vi "MultiTool-Track-Generate-ndipolarisFileOutput-Q-vectors-Accepts Joystick Command with Time Display-Testing time diff with tick-26Apr2017.vi"() -> ()   [LabVIEW 2013]
panel:
  out "TIME":string
  out "bytes written":i32
  out "Return time string":string
  out "Length":u8
  out "Command":u8
  out "Tool 2":T1={"Port Handle"="", "Frame Number"=0, "Tx"=0.0, "Ty"=0.0, "Tz"=0.0, "Q0"=0.0, "Qx"=0.0, "Qy"=0.0, "Qz"=0.0, "Deviation"=0.0, " Markers Missing"=TRUE, "Out of Volume"=TRUE} {"Deviation" format="%#.4f"; "Qz" format="%#.4f"; "Qy" format="%#.4f"; "Qx" format="%#.4f"; "Q0" format="%#.4f"; "Tz" format="%#.2f"; "Ty" format="%#.2f"; "Tx" format="%#.2f"}
  in  "Location of ROM File for Tool 2":path=path "C:/Program Files (x86)/Northern Digital Inc/8700339.rom"
  in  "NDI  Running":bool=TRUE
  out "Stop Reading":bool=TRUE
  out "Start Reading":bool
  out "Object Identifier":string="0"
  in  "Track Outside Measurement Volume? (F:No)":bool
  in  "Track Stray Markers? (F:No)":bool
  out "Tool 1":T1={"Port Handle"="", "Frame Number"=0, "Tx"=0.0, "Ty"=0.0, "Tz"=0.0, "Q0"=0.0, "Qx"=0.0, "Qy"=0.0, "Qz"=0.0, "Deviation"=0.0, " Markers Missing"=TRUE, "Out of Volume"=TRUE} {"Deviation" format="%#.4f"; "Qz" format="%#.4f"; "Qy" format="%#.4f"; "Qx" format="%#.4f"; "Q0" format="%#.4f"; "Tz" format="%#.2f"; "Ty" format="%#.2f"; "Tx" format="%#.2f"}
  out "TCP loop":i32
  in  "TCP Server Running":bool=TRUE
  in  "Output Directory":path=path "C:/Users/Diogo/Desktop/NDI-Labview Gripper"
  out "NDI Loop":i32
  in  "VISA resource name":refnum<visa-resource-name>="COM8"
  in  "Reset? (T:Yes)":bool=TRUE
  in  "Location of ROM File for Tool 1":path=path "C:/Program Files (x86)/Northern Digital Inc/8700449.rom"
  in  "Serial Configuration":T2={"Baud Rate (9600)"=9600, "Flow Control (0:None)"=0, "Parity"=0, "Data Bits"=8, "Stop Bits"=10} {"Stop Bits" items=["1.0"=10, "2.0"=20]; "Parity" items=["None", "Odd", "Even"]; "Flow Control (0:None)" items=["None", "XON/XOFF"]; "Baud Rate (9600)" items=["9600"=9600, "14.4k"=14400, "19.2k"=19200, "38.4k"=38400, "57.6k "=57600, "115.2k"=115200]}
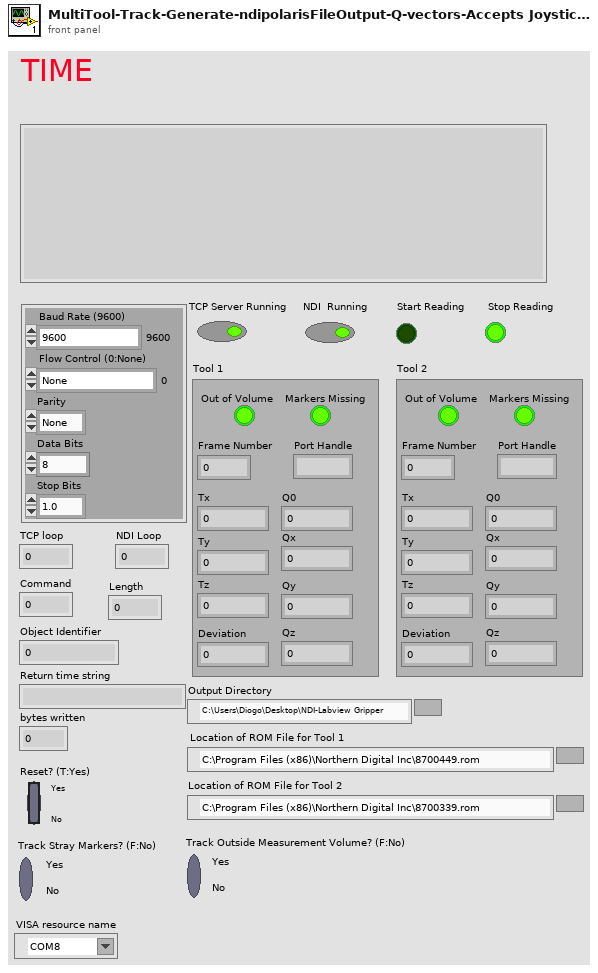
[diagram p1: front panel]
types:
  T1 = cluster{"Port Handle":string, "Frame Number":i32, "Tx":dbl, "Ty":dbl, "Tz":dbl, "Q0":dbl, "Qx":dbl, "Qy":dbl, "Qz":dbl, "Deviation":dbl, " Markers Missing":bool, "Out of Volume":bool}
  T2 = cluster{"Baud Rate (9600)":u32, "Flow Control (0:None)":u16, "Parity":u16, "Data Bits":u16, "Stop Bits":u16}
  T3 = cluster{"Port Handle":string, "Frame Number":u32, "Tx":dbl, "Ty":dbl, "Tz":dbl, "Q0":dbl, "Qx":dbl, "Qy":dbl, "Qz":dbl, "Deviation":dbl, "Missing?":bool, "Out of Volume?":bool}[]
  T4 = cluster{"Transformations[0]":cluster{"Port Handle":string, "Frame Number":u32, "Tx":dbl, "Ty":dbl, "Tz":dbl, "Q0":dbl, "Qx":dbl, "Qy":dbl, "Qz":dbl, "Deviation":dbl, "Missing?":bool, "Out of Volume?":bool}, "Transformations[1]":cluster{"Port Handle":string, "Frame Number":u32, "Tx":dbl, "Ty":dbl, "Tz":dbl, "Q0":dbl, "Qx":dbl, "Qy":dbl, "Qz":dbl, "Deviation":dbl, "Missing?":bool, "Out of Volume?":bool}, "Transformations[2]":cluster{"Port Handle":string, "Frame Number":u32, "Tx":dbl, "Ty":dbl, "Tz":dbl, "Q0":dbl, "Qx":dbl, "Qy":dbl, "Qz":dbl, "Deviation":dbl, "Missing?":bool, "Out of Volume?":bool}, "Transformations[3]":cluster{"Port Handle":string, "Frame Number":u32, "Tx":dbl, "Ty":dbl, "Tz":dbl, "Q0":dbl, "Qx":dbl, "Qy":dbl, "Qz":dbl, "Deviation":dbl, "Missing?":bool, "Out of Volume?":bool}, "Transformations[4]":cluster{"Port Handle":string, "Frame Number":u32, "Tx":dbl, "Ty":dbl, "Tz":dbl, "Q0":dbl, "Qx":dbl, "Qy":dbl, "Qz":dbl, "Deviation":dbl, "Missing?":bool, "Out of Volume?":bool}, "Transformations[5]":cluster{"Port Handle":string, "Frame Number":u32, "Tx":dbl, "Ty":dbl, "Tz":dbl, "Q0":dbl, "Qx":dbl, "Qy":dbl, "Qz":dbl, "Deviation":dbl, "Missing?":bool, "Out of Volume?":bool}, "Transformations[6]":cluster{"Port Handle":string, "Frame Number":u32, "Tx":dbl, "Ty":dbl, "Tz":dbl, "Q0":dbl, "Qx":dbl, "Qy":dbl, "Qz":dbl, "Deviation":dbl, "Missing?":bool, "Out of Volume?":bool}, "Transformations[7]":cluster{"Port Handle":string, "Frame Number":u32, "Tx":dbl, "Ty":dbl, "Tz":dbl, "Q0":dbl, "Qx":dbl, "Qy":dbl, "Qz":dbl, "Deviation":dbl, "Missing?":bool, "Out of Volume?":bool}, "Transformations[8]":cluster{"Port Handle":string, "Frame Number":u32, "Tx":dbl, "Ty":dbl, "Tz":dbl, "Q0":dbl, "Qx":dbl, "Qy":dbl, "Qz":dbl, "Deviation":dbl, "Missing?":bool, "Out of Volume?":bool}}
  T5 = cluster{"Port Handle":string, "Frame Number":u32, "Tx":dbl, "Ty":dbl, "Tz":dbl, "Q0":dbl, "Qx":dbl, "Qy":dbl, "Qz":dbl, "Deviation":dbl, "Missing?":bool, "Out of Volume?":bool}
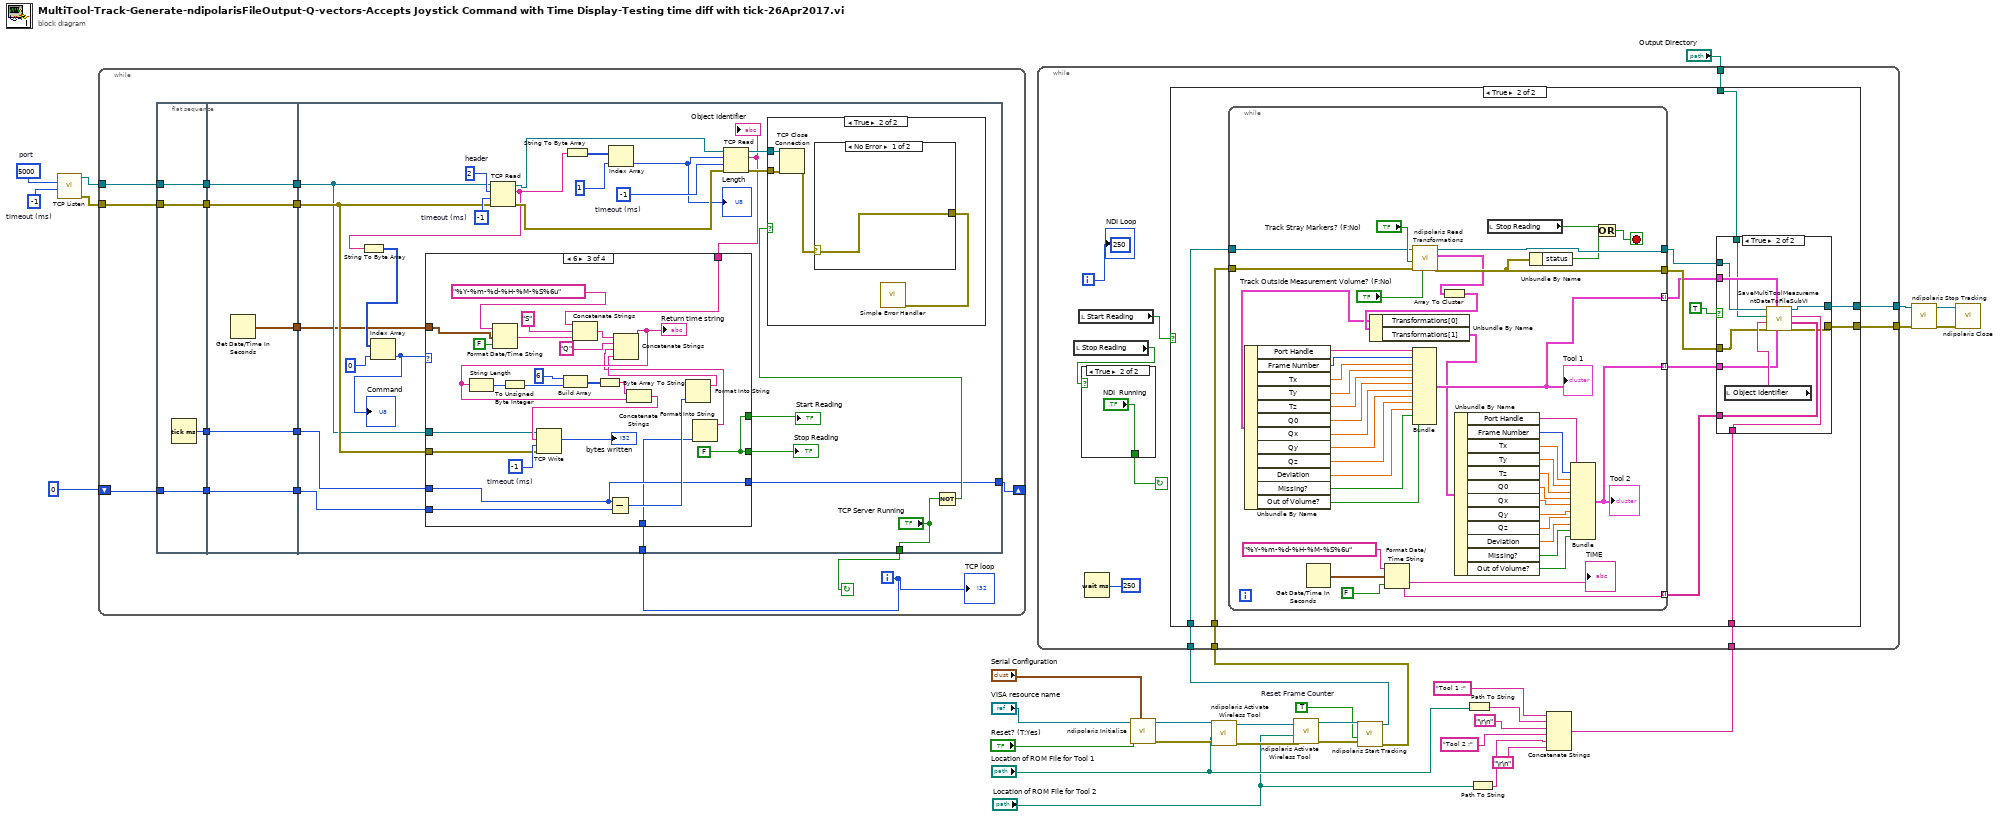
[diagram p0: block diagram]
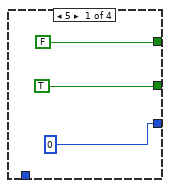
[diagram p2: hidden frame]
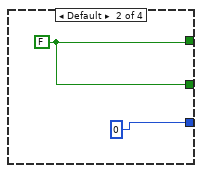
[diagram p3: hidden frame]
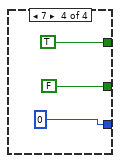
[diagram p4: hidden frame]
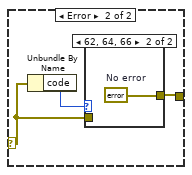
[diagram p6: hidden frame]
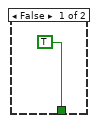
[diagram p8: hidden frame]
diagram:
  w22 = TRUE  # Reset Frame Counter
  w31 = u16 5000  # port
  w30 = i8 -1  # timeout (ms)
  n1 = call <vilib>:"TCP Listen.vi"("timeout ms (wait forever: -1)"=w30, "port"=w31) -> ("error out"=w25:errorcluster, "connection ID"=w26:refnum<k5>)  [unwired: 5 in, 3 out]
  n2 = while {
    tunnel: w26 -> [w44]
    tunnel: w25 -> [w45]
    shift-right: [w38] -> _
    shift-left: u32 0 -> [w40]
    i -> [w32]
    stop <- w46 continue-if-true
    n3 = flat-sequence {
      tunnel: w40 -> [w48]
      tunnel: w44 -> [w49]
      tunnel: w45 -> [w50]
      tunnel: [w50] -> w37
      tunnel: [w49] -> w36
      tunnel: [w48] -> w35
      tunnel: [w47] -> w33
      tunnel: [w55] -> w43
      tunnel: [w54] -> w42
      tunnel: [w53] -> w41
      tunnel: [w52] -> w39
      tunnel: w37 -> [w55]
      tunnel: w36 -> [w54]
      tunnel: w35 -> [w52]
      tunnel: [w51] -> w34
      tunnel: w33 -> [w51]
      tunnel: ["TCP Server Running"] -> w46
      tunnel: w43 -> [w63]
      tunnel: w42 -> [w61]
      tunnel: w41 -> [w60]
      tunnel: w39 -> [w59]
      tunnel: [w58] -> w38
      tunnel: w34 -> [w57]
      tunnel: w32 -> [w56]
      frame #0 {
        n4 = Tick Count (ms)() -> (millisecond timer value=w47:u32)
      }
      frame #1 {
        n5 = Get Date/Time In Seconds() -> (seconds since 1Jan1904=w53:timestamp)
      }
      frame #2 {
        w77 = i8 -1  # timeout (ms)
        w80 = i8 -1  # timeout (ms)
        w81 = i8 2  # header
        n6 = TCP Read(connection ID=w61, bytes to read=w81, error in (no error)=w63, 9:w80) -> (connection ID out=w79:refnum<k5>, data out=w68:string, error out=w78:errorcluster)  [unwired: 1 in]
        n7 = String To Byte Array(string=w68) -> (unsigned byte array=w71:u8[])
        n8 = Index Array(array=w71, index=0) -> (element=w64:u8)
        "Command" <- w64
        n9 = String To Byte Array(string=w68) -> (unsigned byte array=w70:u8[])
        n10 = Index Array(array=w70, index=1) -> (element=w67:u8)
        "Length" <- w67
        n11 = TCP Read(connection ID=w79, bytes to read=w67, error in (no error)=w78, 9:w77) -> (connection ID out=w76:refnum<k5>, data out=w62:string, error out=w75:errorcluster)  [unwired: 1 in]
        "Object Identifier" <- w62
        n12 = case shown="6" w64 {
          tunnel: [FALSE w86 w98 TRUE] -> w74
          tunnel: [TRUE w86 w98 FALSE] -> w73
          tunnel: w63 -> [_ _ w101 _]
          tunnel: w62 -> [_ _ w100 _]
          tunnel: w61 -> [_ _ w99 _]
          tunnel: w60 -> [_ _ w97 _]
          tunnel: w59 -> [_ _ w91 _]
          tunnel: [u32 0 u32 0 w90 u32 0] -> w58
          tunnel: w57 -> [_ _ w90 _]
          tunnel: w56 -> [_ _ w87 _]
          frame 5 {
          }
          frame Default {
            w86 = FALSE
          }
          frame 6 {
            w109 = i8 -1  # timeout (ms)
            w98 = FALSE
            n13 = Format Date/Time String(time format string (%c)="%Y-%m-%d-%H-%M-%S%6u", seconds (now)=w97, UTC format=FALSE) -> (date/time string=w112:string)
            n14 = Concatenate Strings(w100, "S", w112) -> (w96:string)
            n15 = Subtract(x=w90, y=w91) -> (x-y=w92:u32)
            n16 = Format Into String(w92) -> (resulting string=w89:string)  [unwired: 3 in, 1 out]
            n17 = Format Into String(w87) -> (resulting string=w88:string)  [unwired: 3 in, 1 out]
            n18 = Concatenate Strings(w96, "Q", w88, w89) -> (w94:string)
            "Return time string" <- w94
            n19 = String Length(string=w94) -> (length=w106:i32)
            n20 = To Unsigned Byte Integer(number=w106) -> (unsigned 8bit integer=w105:u8)
            n21 = Build Array(u8 6, w105) -> (w103:u8[])
            n22 = Byte Array To String(unsigned byte array=w103) -> (string=w108:string)
            n23 = Concatenate Strings(w108, w94) -> (w102:string)
            n24 = TCP Write(connection ID=w99, data in=w102, error in (no error)=w101, 9:w109) -> (bytes written=→"bytes written":i32)  [unwired: 2 out]
          }
          frame 7 {
          }
        }
        "Start Reading" <- w74
        "Stop Reading" <- w73
        n25 = Not(x="TCP Server Running") -> (.not. x?=w65:bool)
        n26 = case shown="True" w65 {
          tunnel: w76 -> [_ w117]
          tunnel: w75 -> [_ w116]
          frame False {
          }
          frame True {
            n27 = TCP Close Connection(connection ID=w117, error in (no error)=w116) -> (error out=w118:errorcluster)  [unwired: 1 in, 1 out]
            n28 = case shown="No Error" w118 {
              selector: w118 -> [w120 w122]
              tunnel: [w120 w121] -> w119
              frame No Error {
              }
              frame Error {
                n29 = Unbundle By Name(w122) -> ("code"=w123:i32)
                n30 = case shown="62, 64, 66" w123 {
                  tunnel: w122 -> [w124 _]
                  tunnel: [w124 w125] -> w121
                  frame Default {
                  }
                  frame 62, 64, 66 {
                    w125 = errorcluster {"status"=FALSE, "code"=0, "source"=""}  # No error
                  }
                }
              }
            }
            n31 = call <vilib>:"Simple Error Handler.vi"("error in (no error)"=w119) -> ()  [unwired: 1 in, 8 out]
          }
        }
      }
    }
    "TCP loop" <- w32
  }
  n32 = call <instrlib>:"ndipolaris Initialize.vi"("Serial Configuration"="Serial Configuration", "Reset? (T: Yes)"="Reset? (T:Yes)", "VISA resource name"="VISA resource name") -> ("error out"=w12:errorcluster, "VISA resource name out"=w13:refnum<visa-resource-name>)  [unwired: 7 in]
  n33 = call <instrlib>:"ndipolaris Activate Wireless Tool.vi"("error in (no error)"=w12, "Location of ROM File for Tool"="Location of ROM File for Tool 1", "VISA resource name"=w13) -> ("error out"=w10:errorcluster, "VISA resource out"=w11:refnum<visa-resource-name>)  [unwired: 6 in, 1 out]
  n34 = call <instrlib>:"ndipolaris Activate Wireless Tool.vi"("error in (no error)"=w10, "Location of ROM File for Tool"="Location of ROM File for Tool 2", "VISA resource name"=w11) -> ("error out"=w23:errorcluster, "VISA resource out"=w24:refnum<visa-resource-name>)  [unwired: 6 in, 1 out]
  n35 = call <instrlib>:"ndipolaris Start Tracking.vi"("error in (no error)"=w23, "Reset Frame Counter? (F:No)"=w22, "VISA resource name"=w24) -> ("error out"=w17:errorcluster, "VISA resource out"=w21:refnum<visa-resource-name>)  [unwired: 7 in]
  n36 = Path To String(path="Location of ROM File for Tool 1") -> (string=w6:string)
  n37 = Path To String(path="Location of ROM File for Tool 2") -> (string=w4:string)
  n38 = Concatenate Strings("Tool 1 :" ("string"), w6, "\r\n", "Tool 2 :" ("string"), w4, "\r\n") -> (w14:string)
  n39 = while {
    tunnel: w21 -> [w135]
    tunnel: [w134] -> w18
    tunnel: w17 -> [w133]
    tunnel: "Output Directory" -> [w132]
    tunnel: [w131] -> w15
    tunnel: w14 -> [w127]
    i -> [w136]
    stop <- w126 continue-if-true
    (unwired) u8 250
    n40 = local read "Stop Reading"() -> (w128:bool)
    n41 = local read "Start Reading"() -> (w129:bool)
    n42 = case shown="True" w128 {
      tunnel: [TRUE "NDI  Running"] -> w126
      frame False {
      }
      frame True {
      }
    }
    n43 = Wait (ms)(milliseconds to wait=u32 250) -> ()  [unwired: 1 out]
    n44 = case shown="True" w129 {
      tunnel: w135 -> [w140 w152]
      tunnel: [w140 w148] -> w134
      tunnel: w133 -> [w139 w151]
      tunnel: w132 -> [_ w150]
      tunnel: [w139 w147] -> w131
      tunnel: w127 -> [_ w142]
      frame False {
      }
      frame True {
        n45 = while {
          tunnel: [w206] -> w144
          tunnel: [w205] -> w149
          tunnel: [w182] -> w145 mode=indexing
          tunnel: [w183] -> w146 mode=indexing
          tunnel: w152 -> [w181]
          tunnel: w151 -> [w180]
          tunnel: [w165] -> w141 mode=indexing
          stop <- w207 stop-if-true
          n46 = Get Date/Time In Seconds() -> (seconds since 1Jan1904=w186:timestamp)
          n47 = Format Date/Time String(time format string (%c)="%Y-%m-%d-%H-%M-%S%6u", seconds (now)=w186, UTC format=FALSE) -> (date/time string=w183:string)
          "TIME" <- w183
          n48 = call <instrlib>:"ndipolaris Read Transformations.vi"("Track Outside Measurement Volume? (F:No)"="Track Outside Measurement Volume? (F:No)", "error in (no error)"=w180, "Track Stray Markers? (F:No)"="Track Stray Markers? (F:No)", "VISA resource name"=w181) -> ("error out"=w205:errorcluster, "Transformations"=w190:T3, "VISA resource out"=w206:refnum<visa-resource-name>)  [unwired: 4 in, 1 out]
          n49 = Array To Cluster(array=w190) -> (cluster=w201:T4)
          n50 = Unbundle By Name(w201) -> ("Transformations[0]"=w200:T5, "Transformations[1]"=w178:T5)
          n51 = Unbundle By Name(w200) -> ("Port Handle"=w199:string, "Frame Number"=w198:u32, "Tx"=w197:dbl, "Ty"=w196:dbl, "Tz"=w195:dbl, "Q0"=w194:dbl, "Qx"=w193:dbl, "Qy"=w192:dbl, "Qz"=w191:dbl, "Deviation"=w189:dbl, "Missing?"=w188:bool, "Out of Volume?"=w187:bool)
          n52 = Bundle("Port Handle"=w199, "Frame Number"=w198, "Tx"=w197, "Ty"=w196, "Tz"=w195, "Q0"=w194, "Qx"=w193, "Qy"=w192, "Qz"=w191, "Deviation"=w189, "Missing?"=w188, "Out of Volume?"=w187) -> (w182:T5)  [unwired: 1 in]
          "Tool 1" <- w182
          n53 = Unbundle By Name(w178) -> ("Port Handle"=w177:string, "Frame Number"=w176:u32, "Tx"=w175:dbl, "Ty"=w174:dbl, "Tz"=w173:dbl, "Q0"=w172:dbl, "Qx"=w171:dbl, "Qy"=w170:dbl, "Qz"=w169:dbl, "Deviation"=w168:dbl, "Missing?"=w167:bool, "Out of Volume?"=w166:bool)
          n54 = local read "Stop Reading"() -> (w179:bool)
          n55 = Unbundle By Name(w205) -> ("status"=w204:bool)
          n56 = Bundle("Port Handle"=w177, "Frame Number"=w176, "Tx"=w175, "Ty"=w174, "Tz"=w173, "Q0"=w172, "Qx"=w171, "Qy"=w170, "Qz"=w169, "Deviation"=w168, "Missing?"=w167, "Out of Volume?"=w166) -> (w165:T5)  [unwired: 1 in]
          "Tool 2" <- w165
          n57 = Or(x=w179, y=w204) -> (x .or. y?=w207:bool)
        }
        n58 = case shown="True" TRUE {
          tunnel: w150 -> [_ w162]
          tunnel: w149 -> [w153 w160]
          tunnel: [w154 w159] -> w148
          tunnel: [w153 w155] -> w147
          tunnel: w146 -> [_ w158]
          tunnel: w145 -> [_ w164]
          tunnel: w144 -> [w154 w163]
          tunnel: w142 -> [_ w157]
          tunnel: w141 -> [_ w156]
          frame False {
          }
          frame True {
            n59 = local read "Object Identifier"() -> (w161:string)
            n60 = call "SaveMultiToolMeasurementDataToFileSubVI.vi"("Array of Time for Measurement"=w158, "NDI Tool"=w157, "Array - Transformations of Tool 2"=w156, "Array - Transformations of Tool 1"=w164, "error in (no error)"=w160, "Object number"=w161, "Output Directory"=w162, "VISA Refnum in"=w163) -> ("error out"=w155:errorcluster, "VISA Refnum out"=w159:refnum<visa-resource-name>)
          }
        }
      }
    }
    "NDI Loop" <- w136
  }
  n61 = call <instrlib>:"ndipolaris Stop Tracking.vi"("error in (no error)"=w15, "VISA resource name"=w18) -> ("error out"=w19:errorcluster, "VISA resource out"=w20:refnum<visa-resource-name>)  [unwired: 8 in]
  n62 = call <instrlib>:"ndipolaris Close.vi"("error in (no error)"=w19, "VISA resource name"=w20) -> ()  [unwired: 9 in, 1 out]
